vi "DHE_SyncImage.vi"() -> (2 "cmds2exec":string[](array[string]))   [LabVIEW 2016]
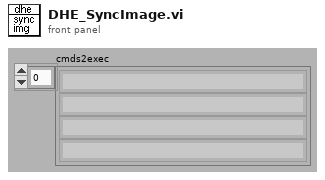
[diagram p1: front panel]
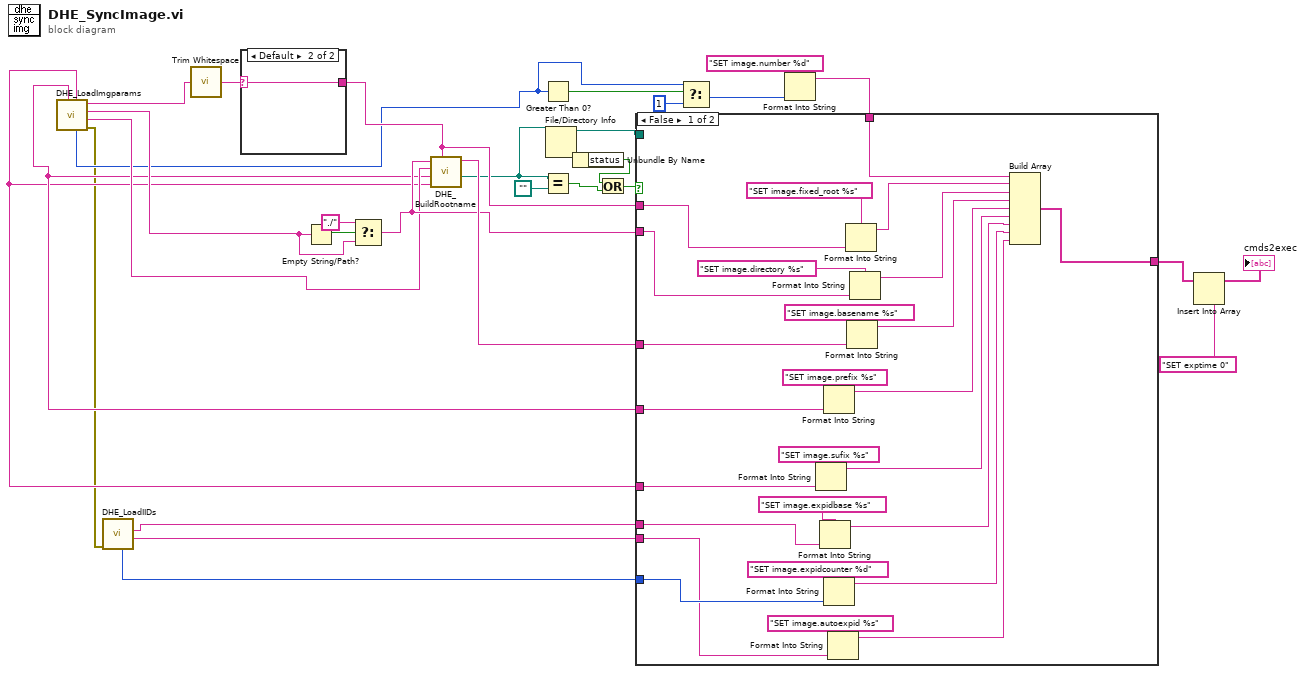
[diagram p0: block diagram]
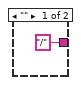
[diagram p2: hidden frame]
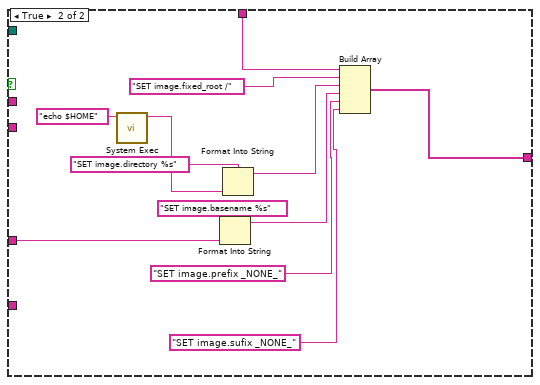
[diagram p3: hidden frame]
diagram:
  n1 = call "DHE_LoadImgparams.vi"() -> ("error out"=w4:errorcluster, "basename"=w14:string, "dir"=w15:string, "froot"=w16:string, "number"=w13:i32, "sufix"=w11:string, "prefix"=w12:string)  [unwired: 1 in, 4 out]
  n2 = call "DHE_LoadIIDs.vi"("error in (no error)"=w4) -> ("autoid"=w2:string, "expidbase"=w3:string, "expidcounter"=w1:i32)  [unwired: 8 out]
  n3 = call <vilib>:"Trim Whitespace.vi"("string"=w16) -> ("trimmed string"=w20:string)  [unwired: 1 in]
  n4 = case shown="Default" w20 {
    selector: w20 -> [_ w33]
    tunnel: ["/" w33] -> w21
    frame "" {
    }
    frame Default {
    }
  }
  n5 = Empty String/Path?(string/path=w15) -> (empty?=w24:bool)
  n6 = Select(t="./", s=w24, f=w15) -> (s? t:f=w23:string)
  n7 = call "DHE_BuildRootname.vi"("froot"=w21, "sufix"=w11, "prefix"=w12, "basename"=w14, "imdir"=w23) -> ("rootpath"=w10:path, "basename out"=w25:string)  [unwired: 1 in, 3 out]
  n8 = Greater Than 0?(x=w13) -> (x > 0?=w29:bool)
  n9 = Equal?(x=w10, y=path "") -> (x = y?=w6:bool)
  n10 = File/Directory Info(path=w10) -> (path out=w31:path, error out=w8:errorcluster)  [unwired: 1 in, 5 out]
  n11 = Unbundle By Name(w8) -> ("status"=w7:bool)
  n12 = Or(x=w7, y=w6) -> (x .or. y?=w5:bool)
  n13 = Select(t=w13, s=w29, f=1) -> (s? t:f=w27:i32)
  n14 = Format Into String(format string="SET image.number %d", w27) -> (resulting string=w26:string)  [unwired: 2 in, 1 out]
  n15 = case shown="False" w5 {
    tunnel: w23 -> [w51 _]
    tunnel: w31 -> [_ _]
    tunnel: w26 -> [w56 w70]
    tunnel: [w57 w71] -> w18
    tunnel: w21 -> [w55 _]
    tunnel: w25 -> [w52 w67]
    tunnel: w12 -> [w46 _]
    tunnel: w11 -> [w45 _]
    tunnel: w3 -> [w39 _]
    tunnel: w2 -> [w37 _]
    tunnel: w1 -> [w38 _]
    frame False {
      n16 = Format Into String(format string="SET image.sufix %s", w45) -> (resulting string=w43:string)  [unwired: 2 in, 1 out]
      n17 = Format Into String(format string="SET image.expidbase %s", w39) -> (resulting string=w36:string)  [unwired: 2 in, 1 out]
      n18 = Format Into String(format string="SET image.prefix %s", w46) -> (resulting string=w44:string)  [unwired: 2 in, 1 out]
      n19 = Format Into String(format string="SET image.expidcounter %d", w38) -> (resulting string=w35:string)  [unwired: 2 in, 1 out]
      n20 = Format Into String(format string="SET image.autoexpid %s", w37) -> (resulting string=w34:string)  [unwired: 2 in, 1 out]
      n21 = Format Into String(format string="SET image.fixed_root %s", w55) -> (resulting string=w58:string)  [unwired: 2 in, 1 out]
      n22 = Format Into String(format string="SET image.basename %s", w52) -> (resulting string=w49:string)  [unwired: 2 in, 1 out]
      n23 = Format Into String(format string="SET image.directory %s", w51) -> (resulting string=w50:string)  [unwired: 2 in, 1 out]
      n24 = Build Array(w56, w58, w50, w49, w44, w43, w36, w35, w34) -> (w57:string[])
    }
    frame True {
      n25 = call <vilib>:"System Exec.vi"("command line"="echo $HOME") -> ("standard output"=w62:string)  [unwired: 5 in, 5 out]
      n26 = Format Into String(format string="SET image.basename %s", w67) -> (resulting string=w65:string)  [unwired: 2 in, 1 out]
      n27 = Format Into String(format string="SET image.directory %s", w62) -> (resulting string=w66:string)  [unwired: 2 in, 1 out]
      n28 = Build Array(w70, "SET image.fixed_root /" ("format string"), w66, w65, "SET image.prefix _NONE_" ("format string"), "SET image.sufix _NONE_" ("format string")) -> (w71:string[])
    }
  }
  n29 = Insert Into Array(array=w18, new element="SET exptime 0" ("new element/subarray")) -> (→"cmds2exec":string[])  [unwired: 1 in]
